vi "Match_loop.vi"(1 "No Of Strings":i32, 2 "Match string":string[](array[string]), 3 "Ch Name":string) -> (0 "Matched?":bool)   [LabVIEW 2010]
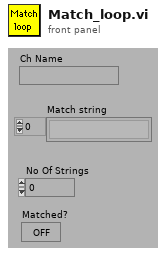
[diagram p1: front panel]
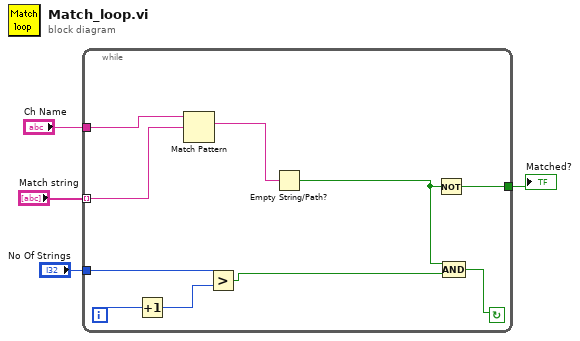
[diagram p0: block diagram]
diagram:
  n1 = while {
    tunnel: [w5] -> w1
    tunnel: "No Of Strings" -> [w11]
    tunnel: "Match string" -> [w13] mode=indexing
    tunnel: "Ch Name" -> [w14]
    i -> [w12]
    stop <- w7 continue-if-true
    n2 = Increment(x=w12) -> (x+1=w10:i32)
    n3 = Match Pattern(string=w14, regular expression=w13) -> (match substring=w9:string)  [unwired: 1 in, 3 out]
    n4 = Greater?(x=w11, y=w10) -> (0:w8:bool)
    n5 = Empty String/Path?(string/path=w9) -> (empty?=w6:bool)
    n6 = Not(x=w6) -> (.not. x?=w5:bool)
    n7 = Compound Arithmetic op=AND(w6, w8) -> (w7:bool)
  }
  "Matched?" <- w1
